vi "TagMotor.vi"(2 "PI Number":enum16{"1", "2"}(ring), 3 "Motor":string, 9 "error in":errorcluster caption="error in (no error)") -> (0 "Tagged Motor":string, 6 "error out":errorcluster)   [LabVIEW 2009]
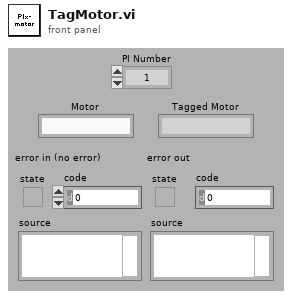
[diagram p1: front panel]
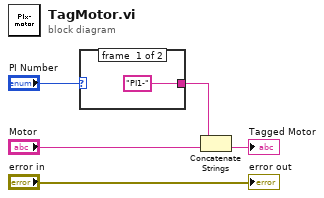
[diagram p0: block diagram]
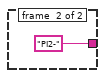
[diagram p2: hidden frame]
diagram:
  n1 = case shown="\"1\", Default" "PI Number" {
    tunnel: ["PI1-" ("Chaîne") "PI2-" ("Chaîne")] -> w4
    frame #0 {
    }
    frame #1 {
    }
  }
  n2 = Concatenate Strings(w4, "Motor") -> (→"Tagged Motor":string)
  "error out" <- "error in"
